vi "ADCMT6240ACtrlProto.vi"() -> ()   [LabVIEW 2017]
uses:
  6240AData.lvclass
panel:
  out "error out":errorcluster
  in  "Voltage limits (V)":dbl[](array[numeric])=[12.0, 12.0]
  out "ActualCurrent (A)":dbl[](array[numeric])
  in  "InstName":string
  in  "RunName":string
  in  "Initialize":bool
  in  "VISA":refnum<visa-resource-name>[](array[refnum])
  in  "base path":path
  in  "Stop Button":bool
  out "XY Graph":T1(graph)
  in  "Output status":bool[](array[boolean])
  in  "SetCurrent (A)":dbl[](array[numeric])
  in  "CtrlLabels":string[](array[string])
  out "Initialized?":bool=TRUE
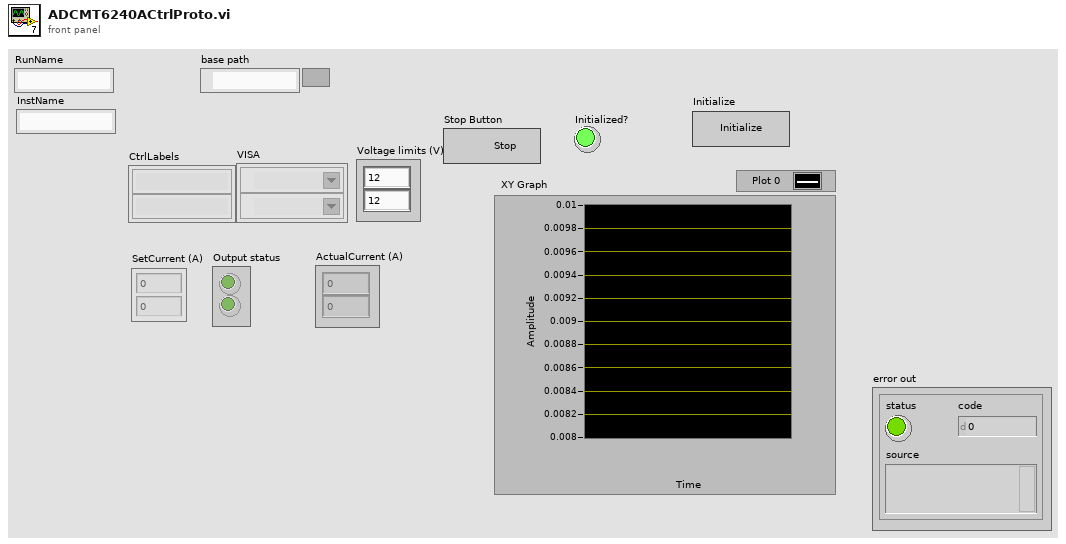
[diagram p1: front panel]
types:
  T1 = cluster{"appended array":timestamp[], "ActualCurrentArray":dbl[]}[]
  T2 = cluster{"appended array":timestamp[], "ActualCurrentArray":dbl[]}
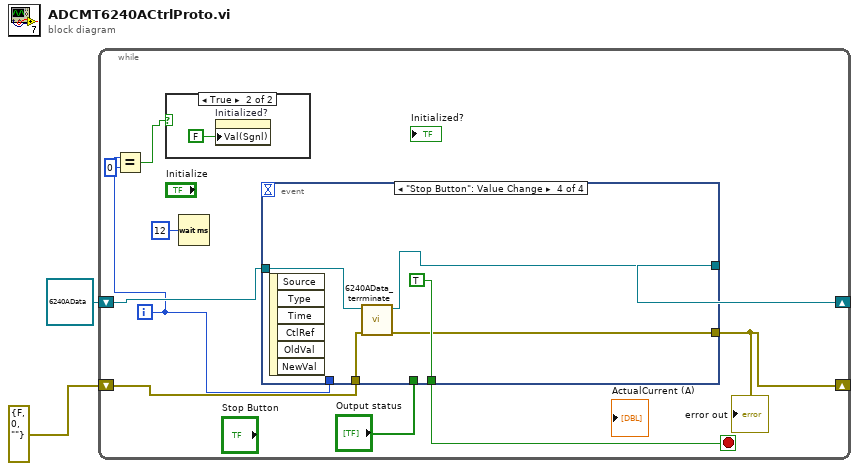
[diagram p0: block diagram]
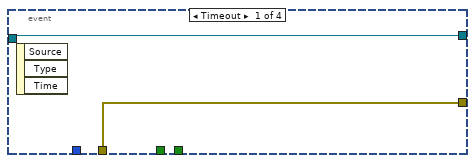
[diagram p3: hidden frame]
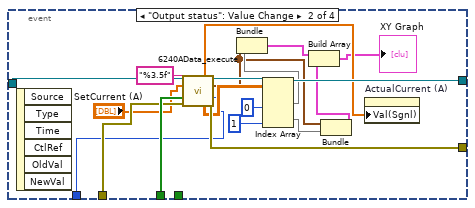
[diagram p4: hidden frame]
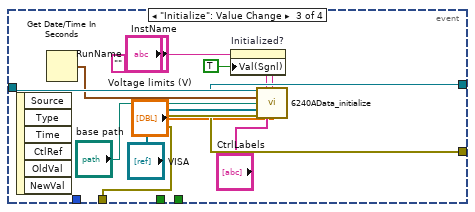
[diagram p5: hidden frame]
diagram:
  n1 = while {
    shift-right: [w12] -> _
    shift-left: refnum<class "6240AData.lvclass"> refnum ("6240AData.lvclass") -> [w9]
    shift-right: [w6] -> _
    shift-left: errorcluster {"status"=FALSE, "code"=0, "source"=""} ("error in (no error)") -> [w8]
    i -> [w5]
    stop <- w10 stop-if-true
    n2 = Equal?(x=w5, y=0) -> (x = y?=w3:bool)
    n3 = case shown="True" w3 {
      frame False {
      }
      frame True {
        n4 = property on="Initialized?" class="Bool (strict)"("Val(Sgnl)"=FALSE ("Value (Signaling)")) -> ()  [unwired: 2 in, 2 out]
      }
    }
    n5 = Wait (ms)(milliseconds to wait=u32 12) -> ()  [unwired: 1 out]
    n6 = event shown="[3] \"Stop Button\": Value Change" {
      selector: _ -> [_ _ _ _]
      dyn-events: _ -> [_ _ _ _]
      timeout: _ -> [_ _ _ _]
      tunnel: [w15 w33 w39 w48] -> w12
      tunnel: "Output status" -> [_ w32 _ _]
      tunnel: [_ _ _ TRUE ("Value (Signaling)")] -> w10
      tunnel: w9 -> [w15 w31 w45 w49]
      tunnel: w8 -> [w14 w30 w41 w47]
      tunnel: [w14 w29 w40 w46] -> w6
      tunnel: w5 -> [_ w22 _ _]
      event Timeout {
        n7 = event-data() -> ()  [unwired: 1 in, 3 out]
      }
      event "Output status": Value Change {
        n8 = event-data() -> ()  [unwired: 1 in, 6 out]
        n9 = call-dynamic "6240AData_execute.vi"("6240AData in"=w31, "SetCurrent (A)"="SetCurrent (A)", "FileFormat"="%3.5f", "Output status"=w32, "ExecutionIndex"=w22, "error in (no error)"=w30) -> ("ActualCurrent (A)"=w21:dbl[], "6240AData out"=w33:refnum<class "6240AData.lvclass">, "appended array"=w19:timestamp[], "ActualCurrentArray"=w27:dbl[][], "error out"=w29:errorcluster)  [unwired: 3 in, 2 out]
        n10 = Index Array(array=w27, index (col) #1=0 ("disabled index (col)"), index (col) #2=1 ("index (col)")) -> (element #1=w28:dbl[], element #2=w18:dbl[])  [unwired: 2 in]
        n11 = Bundle("appended array"=w19, "ActualCurrentArray"=w28) -> (w20:T2)  [unwired: 1 in]
        n12 = Bundle("appended array"=w19, "ActualCurrentArray"=w18) -> (w17:T2)  [unwired: 1 in]
        n13 = Build Array(w20, w17) -> (→"XY Graph":T1)
        n14 = property on="ActualCurrent (A)" class="Arr (strict)"("Val(Sgnl)"=w21) -> ()  [unwired: 2 in, 2 out]
      }
      event "Initialize": Value Change {
        (unwired) "" ("InstName")
        n15 = event-data() -> ()  [unwired: 1 in, 6 out]
        n16 = Get Date/Time In Seconds() -> (seconds since 1Jan1904=w44:timestamp)
        n17 = property on="Initialized?" class="Bool (strict)"("Val(Sgnl)"=TRUE ("Value (Signaling)")) -> ()  [unwired: 2 in, 2 out]
        n18 = call-dynamic "6240AData_initialize.vi"("6240AData in"=w45, "RunName"="RunName", "InstName"="InstName", "start time"=w44, "base path"="base path", "VISA"="VISA", "error in (no error)"=w41, "CtrlLabels"="CtrlLabels", "Voltage limits (V)"="Voltage limits (V)") -> ("6240AData out"=w39:refnum<class "6240AData.lvclass">, "error out"=w40:errorcluster)  [unwired: 5 in]
      }
      event "Stop Button": Value Change {
        n19 = event-data() -> ()  [unwired: 1 in, 6 out]
        n20 = call-dynamic "6240AData_terrminate.vi"("error in (no error)"=w47, "6240AData in"=w49) -> ("error out"=w46:errorcluster, "6240AData out"=w48:refnum<class "6240AData.lvclass">)  [unwired: 8 in]
      }
    }
    "error out" <- w6
  }
